vi "CO 2 Trigger Demo.vi"() -> ()   [LabVIEW 2012]
panel:
  in  "CO2 ppm":dbl(slide) scale=0.0..10000.0 scale format="%#.0f"
  in  "CO2  Trigger":T1={"Boost A Threshold"=3000.0, "Boost A Hyst"=-400.0, "Boost B Threshold"=1400.0, "Boost B Hyst"=-400.0, "Recirc Threshold "=8800.0, "Recirc  Hyst "=-200.0, "O2 Threshold"=9400.0, "O2 Hyst"=-200.0, "Scrubber"=8600.0, "Scrub Hyst"=-200.0, "Vent Threshold"=9000.0, "Vent Hyst"=-200.0, "Alarm Threhols"=9600.0, "Alarm Hyst"=-200.0}
  out "Alt Diff Down":bool=TRUE
  out "CO2 Dif Last":dbl
  in  "Stop Progam":bool
  out "Loops":i32=977
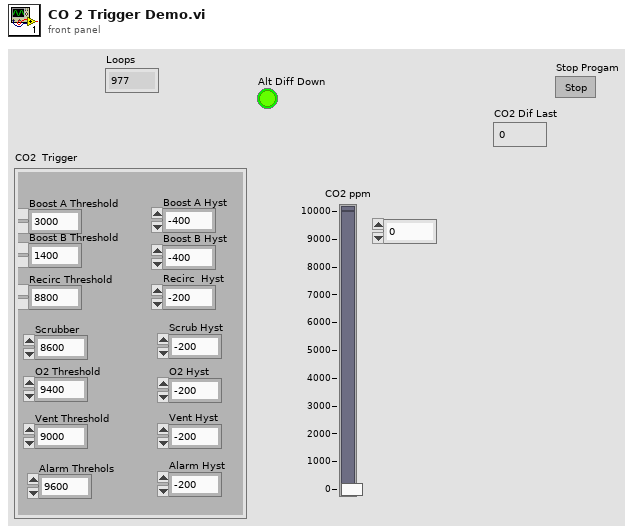
[diagram p1: front panel]
types:
  T1 = cluster{"Boost A Threshold":dbl, "Boost A Hyst":dbl, "Boost B Threshold":dbl, "Boost B Hyst":dbl, "Recirc Threshold ":dbl, "Recirc  Hyst ":dbl, "O2 Threshold":dbl, "O2 Hyst":dbl, "Scrubber":dbl, "Scrub Hyst":dbl, "Vent Threshold":dbl, "Vent Hyst":dbl, "Alarm Threhols":dbl, "Alarm Hyst":dbl}
  T2 = cluster{"Main":bool, "Boost A":bool, "Boost B":bool, "Recirc":bool, "Scrubber":bool, "O2 Valve":bool, "Vent":bool, "Alarm":bool}
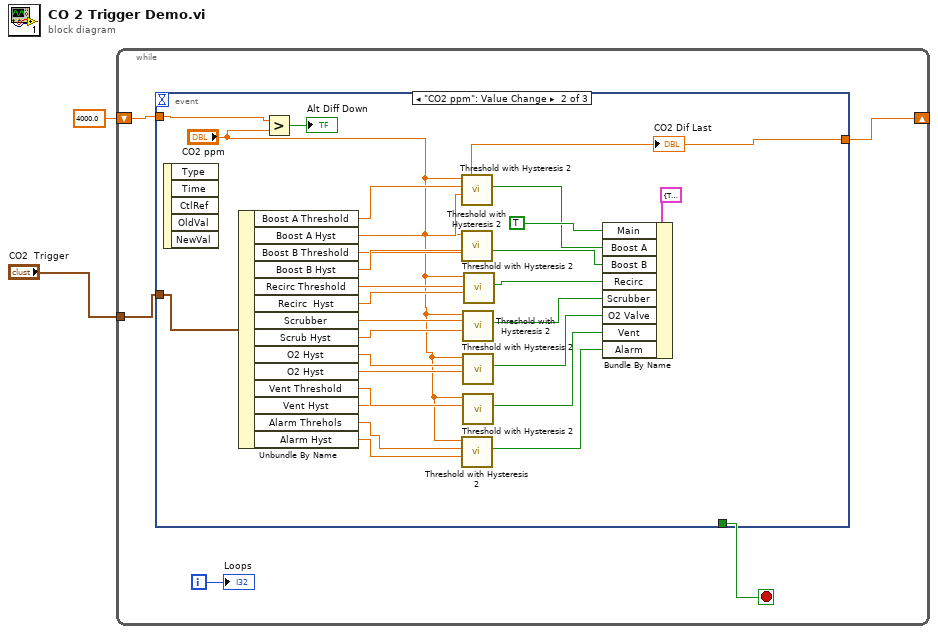
[diagram p0: block diagram]
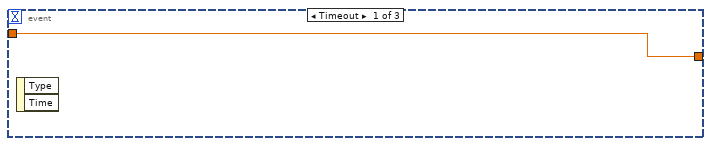
[diagram p2: hidden frame]
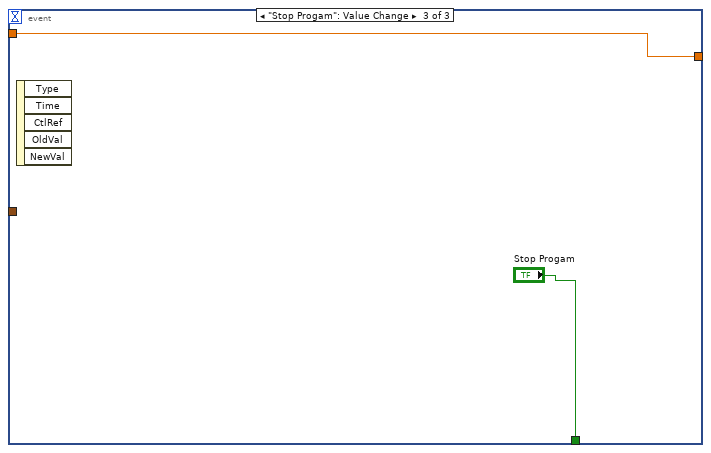
[diagram p3: hidden frame]
diagram:
  n1 = while {
    tunnel: "CO2  Trigger" -> [w7]
    shift-right: [w4] -> _
    shift-left: 4000.0 ("Out Dif Last") -> [w5]
    i -> [w6]
    stop <- w3 stop-if-true
    n2 = event shown="[1] \"CO2 ppm\": Value Change" {
      selector: _ -> [_ _ _]
      dyn-events: _ -> [_ _ _]
      timeout: _ -> [_ _ _]
      tunnel: w7 -> [_ w25 _]
      tunnel: w5 -> [w8 w26 w39]
      tunnel: [w8 w27 w39] -> w4
      tunnel: [_ _ "Stop Progam"] -> w3
      event Timeout {
        n3 = event-data() -> ()  [unwired: 1 in, 2 out]
      }
      event "CO2 ppm": Value Change {
        n4 = event-data() -> ()  [unwired: 1 in, 5 out]
        n5 = Unbundle By Name(w25) -> ("Boost A Threshold"=w34:dbl, "Boost A Hyst"=w33:dbl, "Boost B Threshold"=w30:dbl, "Boost B Hyst"=w31:dbl, "Recirc Threshold"=w24:dbl, "Recirc  Hyst"=w23:dbl, "Scrubber"=w21:dbl, "Scrub Hyst"=w20:dbl, "O2 Hyst"=w19:dbl, "O2 Hyst"=w18:dbl, "Vent Threshold"=w17:dbl, "Vent Hyst"=w16:dbl, "Alarm Threhols"=w14:dbl, "Alarm Hyst"=w13:dbl)
        n6 = Greater?(x=w26, y="CO2 ppm") -> (0:→"Alt Diff Down":bool)
        n7 = call "Threshold with Hysteresis 2.vi"("Hystersis"=w33, "Threshold"=w34, "Input Dif"="CO2 ppm") -> ("Power"=w29:bool, "Out Dif Last"=w27:dbl)  [unwired: 2 in, 2 out]
        "CO2 Dif Last" <- w27
        n8 = call "Threshold with Hysteresis 2.vi"("Hystersis"=w31, "Threshold"=w30, "Input Dif"="CO2 ppm") -> ("Threshold"=w32:bool)  [unwired: 2 in, 3 out]
        n9 = call "Threshold with Hysteresis 2.vi"("Hystersis"=w13, "Threshold"=w14, "Input Dif"="CO2 ppm") -> ("Power"=w9:bool)  [unwired: 2 in, 3 out]
        n10 = call "Threshold with Hysteresis 2.vi"("Hystersis"=w20, "Threshold"=w21, "Input Dif"="CO2 ppm") -> ("Power"=w12:bool)  [unwired: 2 in, 3 out]
        n11 = call "Threshold with Hysteresis 2.vi"("Hystersis"=w18, "Threshold"=w19, "Input Dif"="CO2 ppm") -> ("Power"=w11:bool)  [unwired: 2 in, 3 out]
        n12 = call "Threshold with Hysteresis 2.vi"("Hystersis"=w16, "Threshold"=w17, "Input Dif"="CO2 ppm") -> ("Power"=w10:bool)  [unwired: 2 in, 3 out]
        n13 = call "Threshold with Hysteresis 2.vi"("Hystersis"=w23, "Threshold"=w24, "Input Dif"="CO2 ppm") -> ("Power"=w22:bool)  [unwired: 2 in, 3 out]
        n14 = Bundle By Name(cluster=T2 {"Main"=TRUE, "Boost A"=FALSE, "Boost B"=FALSE, "Recirc"=FALSE, "Scrubber"=FALSE, "O2 Valve"=FALSE, "Vent"=FALSE, "Alarm"=FALSE} ("Alt States"), "Main"=TRUE, "Boost A"=w29, "Boost B"=w32, "Recirc"=w22, "Scrubber"=w12, "O2 Valve"=w11, "Vent"=w10, "Alarm"=w9) -> (w36:T2)
      }
      event "Stop Progam": Value Change {
        n15 = event-data() -> ()  [unwired: 1 in, 5 out]
      }
    }
    "Loops" <- w6
  }
